vi "Handle.vi"(8 "error in (no error)":errorcluster, 10 "Zero Timeout Message Handler in":refnum<class "Zero Timeout Message Handler.lvclass">, 11 "Message in":refnum<class "Get Notifiers Msg.lvclass">) -> (0 "error out":errorcluster, 2 "Zero Timeout Message Handler out":refnum<class "Zero Timeout Message Handler.lvclass">)   [LabVIEW 2024, in "PID Loop.lvlib" / "Get Notifiers Msg.lvclass"]
uses:
  Get Notifiers Msg.lvclass
  Get Notifiers Msg.lvclass/Get Notifiers Msg.ctl
  PID Loop.lvclass
  src/Zero Timeout Message Handler/Zero Timeout Message Handler/Zero Timeout Message Handler.lvclass
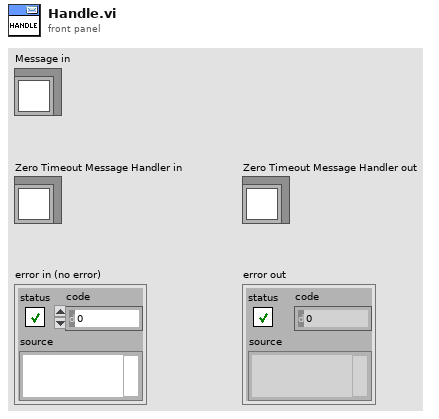
[diagram p1: front panel]
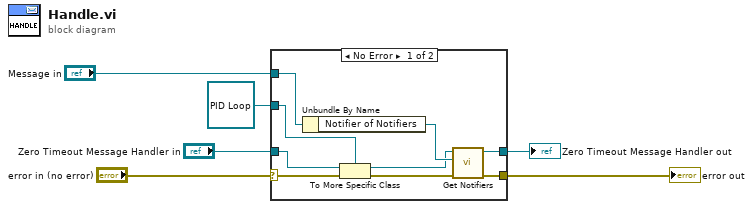
[diagram p0: block diagram]
diagram:
  n1 = case shown="No Error" "error in (no error)" {
    selector: "error in (no error)" -> [w8 w17]
    tunnel: [w15 w16] -> w5
    tunnel: [w14 w17] -> w4
    tunnel: "Message in" -> [w13 _]
    tunnel: refnum<class "PID Loop.lvclass"> refnum ("PID Loop.lvlib:PID Loop.lvclass") -> [w11 _]
    tunnel: "Zero Timeout Message Handler in" -> [w10 w16]
    frame No Error {
      n2 = Unbundle By Name(w13) -> ("Notifier of Notifiers"=w12:refnum<notifier>)
      n3 = To More Specific Class(target class=w11, reference=w10, error in=w8) -> (specific class reference=w9:refnum<class "PID Loop.lvclass">, error out=w7:errorcluster)
      n4 = call-dynamic "Get Notifiers.vi"("error in (no error)"=w7, "Notifier of Notifiers"=w12, "PID Loop in"=w9) -> ("error out"=w14:errorcluster, "PID Loop out"=w15:refnum<class "PID Loop.lvclass">)  [unwired: 7 in]
    }
    frame Error {
    }
  }
  "error out" <- w4
  "Zero Timeout Message Handler out" <- w5
